vi "createPubDataEvents.vi"(8 "error in (no error)":errorcluster, 11 "UserEvents in":refnum<class "UserEvents.lvclass">) -> (0 "error out":errorcluster, 3 "UserEvents out":refnum<class "UserEvents.lvclass">)   [LabVIEW 2013, in "UserEvents.lvclass"]
uses:
  UserEvents.lvclass
  Typedefs/StateSelector.ctl
  Typedefs/InputData.ctl
  Typedefs/ForceSetpoint.ctl
  Typedefs/OutputData.ctl
  Typedefs/ControllerData.ctl
  Typedefs/TestStatus.ctl
  UserEvents.lvclass/UserEvents.ctl
  Typedefs/FAMTTypedefs.lvlib
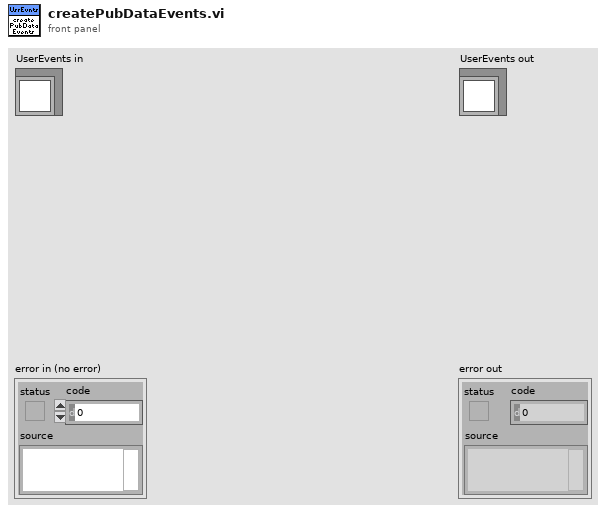
[diagram p1: front panel]
types:
  T1 = typedef "FAMTTypedefs.lvlib/TestStatus.ctl" = cluster{"activeCycle":u32, "activeProfileStep":u32, "demandedCycles":u32, "demandedProfileSteps":u32}
  T2 = typedef "FAMTTypedefs.lvlib/ControllerData.ctl" = cluster{"Force Setpoint":T3, "Force Error":T3}
  T3 = typedef "FAMTTypedefs.lvlib/ForceSetpoint.ctl" = dbl[unit]
  T4 = typedef "FAMTTypedefs.lvlib/OutputData.ctl" = cluster{"Ch1":u16, "Ch2":u16, "Ch3":u16}
  T5 = typedef "FAMTTypedefs.lvlib/InputData.ctl" = cluster{"Force Measured Axial":T3, "Force Measured Lateral":T3}
  T6 = typedef "FAMTTypedefs.lvlib/StateSelector.ctl" = enum16{"EndingCycleState", "FaultState", "InteractiveSetpointState", "OffState", "StandbyState", "StoppedState"}
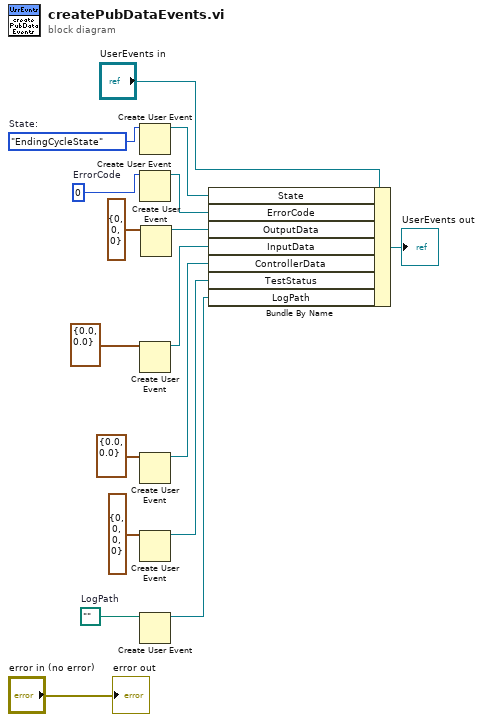
[diagram p0: block diagram]
diagram:
  w2 = path ""  # LogPath
  w13 = 0  # ErrorCode
  w14 = StateSelector."EndingCycleState"  # State:
  n1 = Create User Event(user event datatype=w14) -> (user event=w12:refnum<user-event>)  [unwired: 1 in, 1 out]
  n2 = Create User Event(user event datatype=w13) -> (user event=w11:refnum<user-event>)  [unwired: 1 in, 1 out]
  n3 = Create User Event(user event datatype=T5 {"Force Measured Axial"=0.0, "Force Measured Lateral"=0.0} ("Input Data")) -> (user event=w9:refnum<user-event>)  [unwired: 1 in, 1 out]
  n4 = Create User Event(user event datatype=T2 {"Force Setpoint"=0.0, "Force Error"=0.0} ("Controller Data")) -> (user event=w5:refnum<user-event>)  [unwired: 1 in, 1 out]
  n5 = Create User Event(user event datatype=T1 {"activeCycle"=0, "activeProfileStep"=0, "demandedCycles"=0, "demandedProfileSteps"=0} ("TestStatus")) -> (user event=w3:refnum<user-event>)  [unwired: 1 in, 1 out]
  n6 = Create User Event(user event datatype=w2) -> (user event=w1:refnum<user-event>)  [unwired: 1 in, 1 out]
  n7 = Create User Event(user event datatype=T4 {"Ch1"=0, "Ch2"=0, "Ch3"=0} ("Output Data")) -> (user event=w7:refnum<user-event>)  [unwired: 1 in, 1 out]
  n8 = Bundle By Name(cluster="UserEvents in", "State"=w12, "ErrorCode"=w11, "OutputData"=w7, "InputData"=w9, "ControllerData"=w5, "TestStatus"=w3, "LogPath"=w1) -> (→"UserEvents out":refnum<class "UserEvents.lvclass">)
  "error out" <- "error in (no error)"
